vi "Main.vi"() -> ()   [LabVIEW 2020]
uses:
  Userdata.ctl
  <vilib>/drjdpowell/SQLite Library/SQL Connection/Open (string).vi
  <vilib>/drjdpowell/SQLite Library/SQL Connection/Execute SQL (1D String).vi
  <vilib>/drjdpowell/SQLite Library/SQL Connection/Execute SQL (No results).vi
  <vilib>/drjdpowell/SQLite Library/SQL Connection/Connection.lvclass
  <vilib>/drjdpowell/SQLite Library/SQLite.lvlib
panel:
  in  "Tab Control":T1(tab)
  in  "Login":bool
  in  "Password":string
  in  "Username":string
  in  "Exit 2":bool
  out "?":string
  in  "Add User":bool
  in  "Logout":bool
  in  "Exit":bool
  in  "Edit User":bool
  in  "Query User":bool
  in  "Delete User":bool
  in  "Home Add":bool
  in  "Confirm Add":bool
  in  "Userdata_add_page":T2
  out "?":errorcluster
  in  "Home Delete":bool
  in  "Confirm Delete":bool
  in  "Select User to delete":string(combo)
  out "Userdata_delete_page":T2
  in  "Home query":bool
  in  "Select User to more data":string(combo)
  out "Userdata_Query_page":T2
  in  "Home edit":bool
  in  "Confirm Edit":bool
  in  "Select User to Edit":string(combo)
  in  "Userdata_Edit_page":T2
  out "?":errorcluster
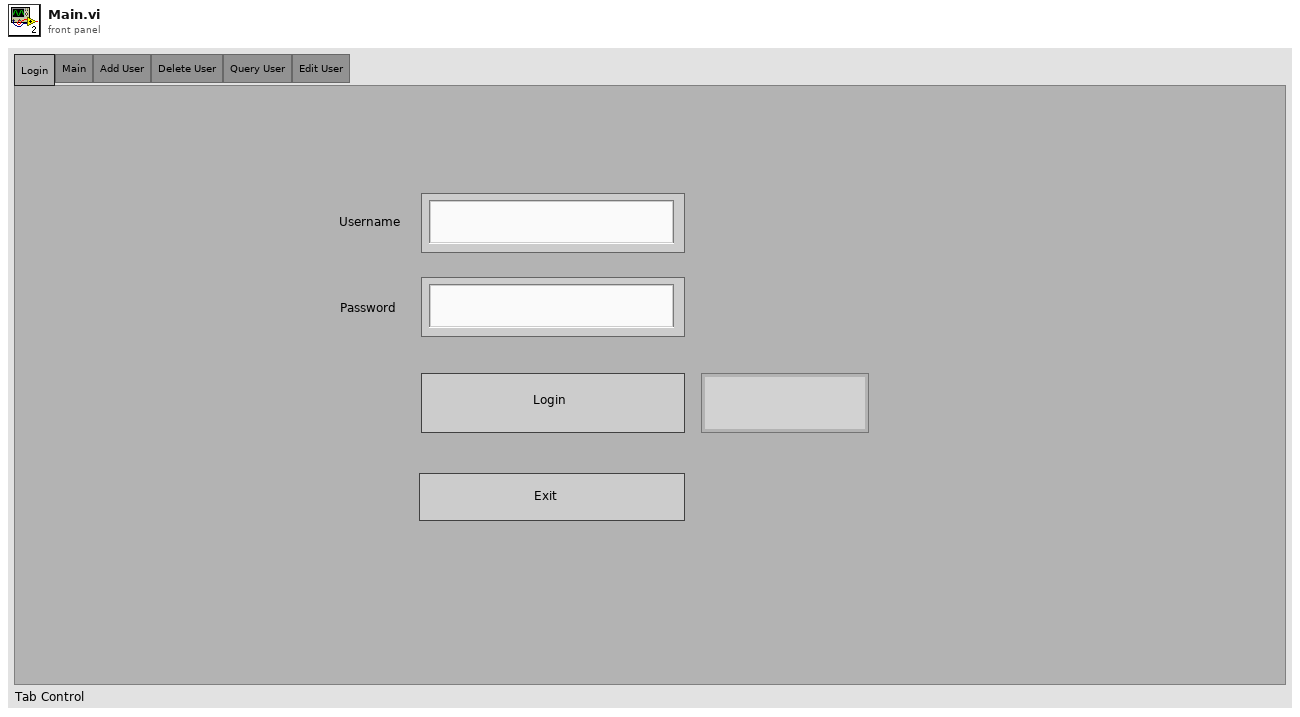
[diagram p1: front panel]
types:
  T1 = enum32{"Login", "Main", "Add User", "Delete User", "Query User", "Edit User"}
  T2 = typedef "Userdata.ctl" = cluster{"Username":string, "Password":string, "Title":string, "Birthdate":timestamp, "Email":string, "User Level":bool}
  T3 = enum32{"Page Enabled", "Page Disabled", "Page Disabled & Grayed"}
  T4 = cluster{"Username":bool, "Password":bool, "Title":bool, "Birthdate":bool, "Email":bool, "User Level":bool}
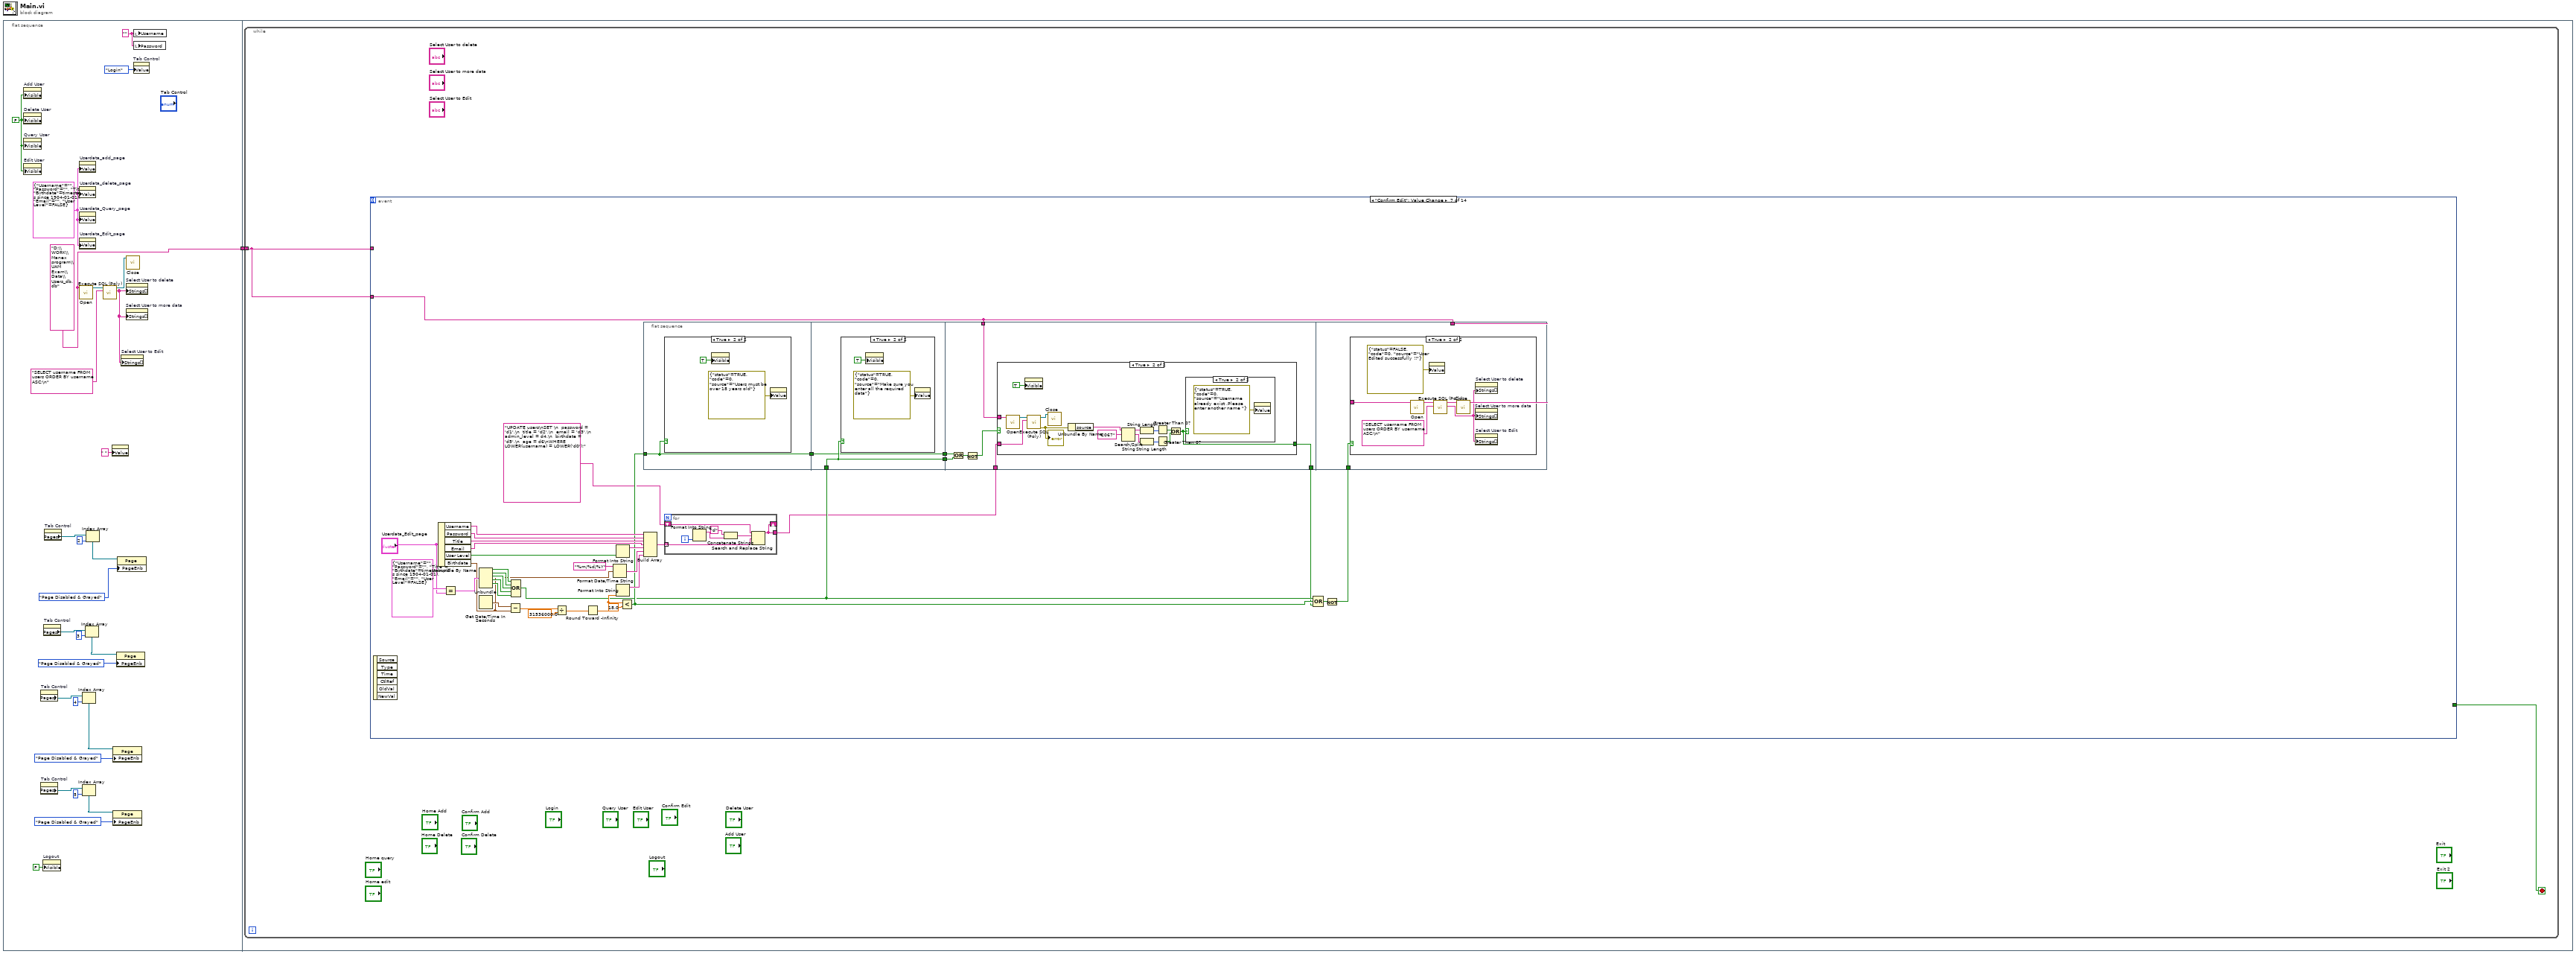
[diagram p0: block diagram]
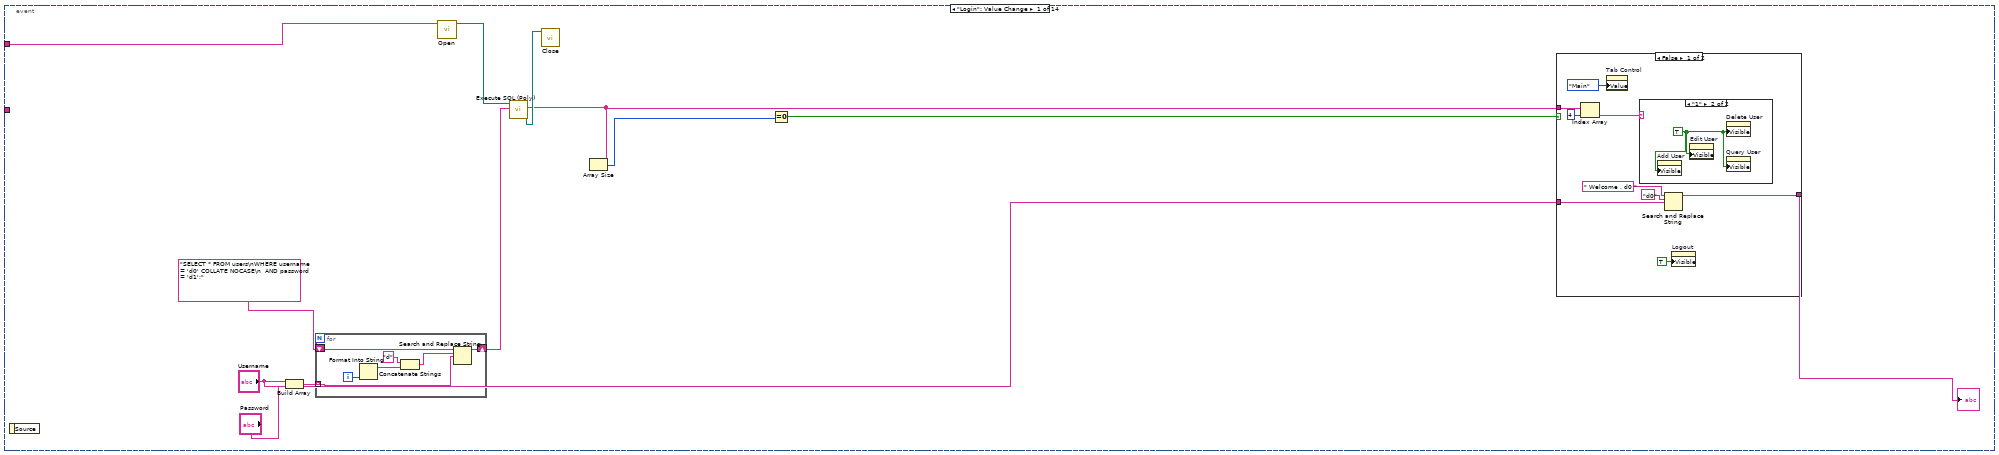
[diagram p2: hidden frame]
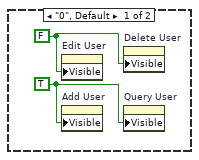
[diagram p3: hidden frame]
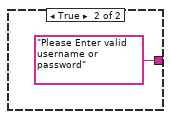
[diagram p4: hidden frame]
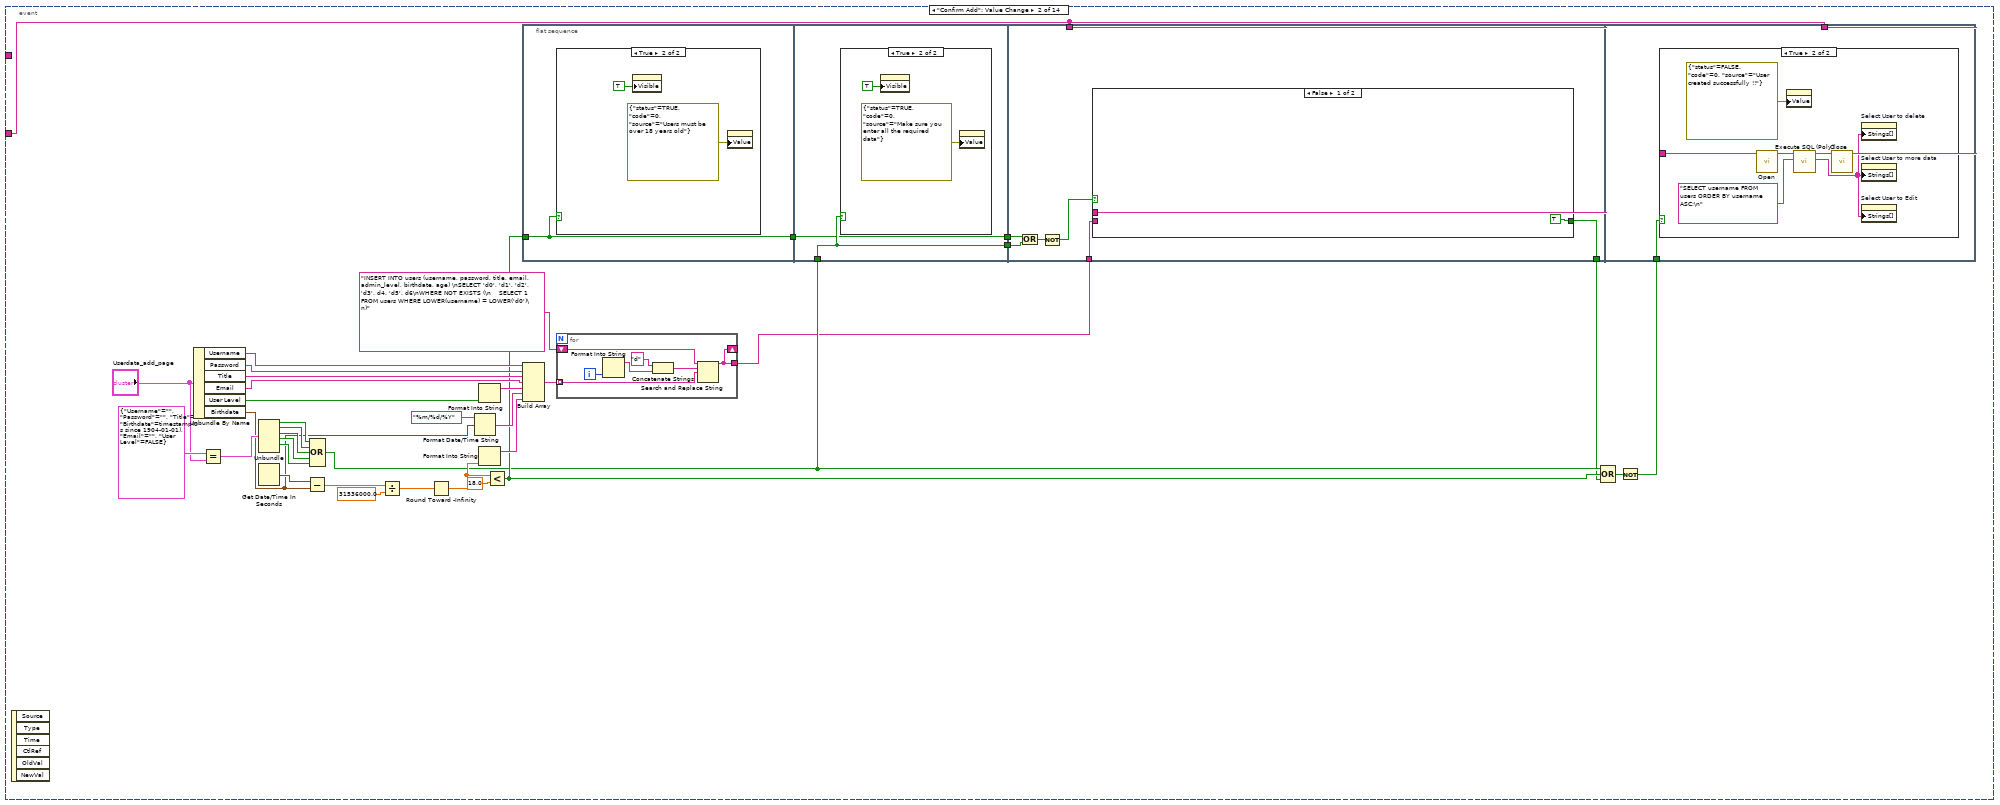
[diagram p5: hidden frame]
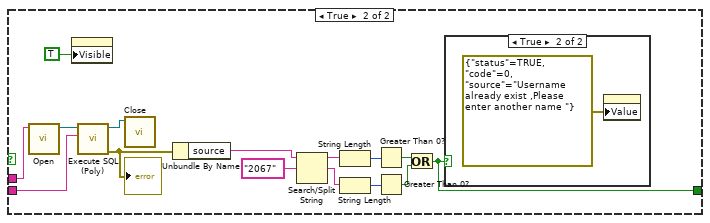
[diagram p8: hidden frame]
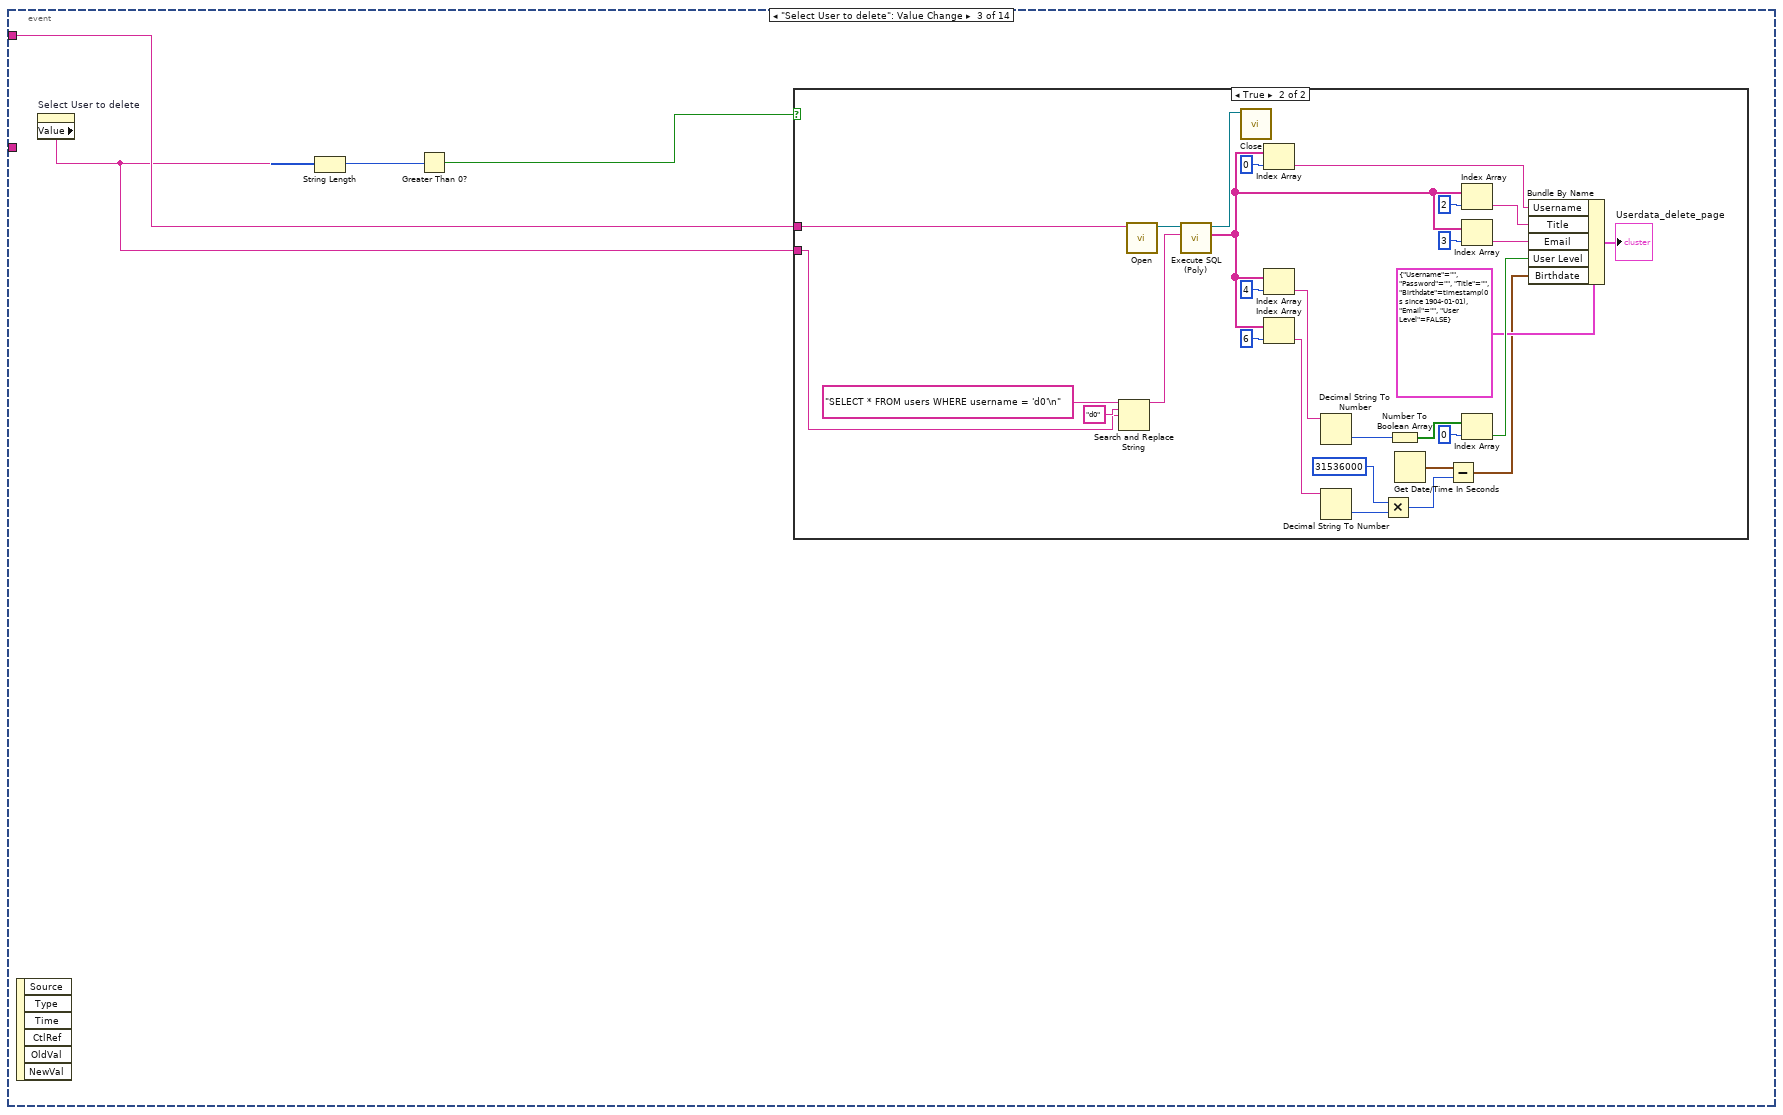
[diagram p11: hidden frame]
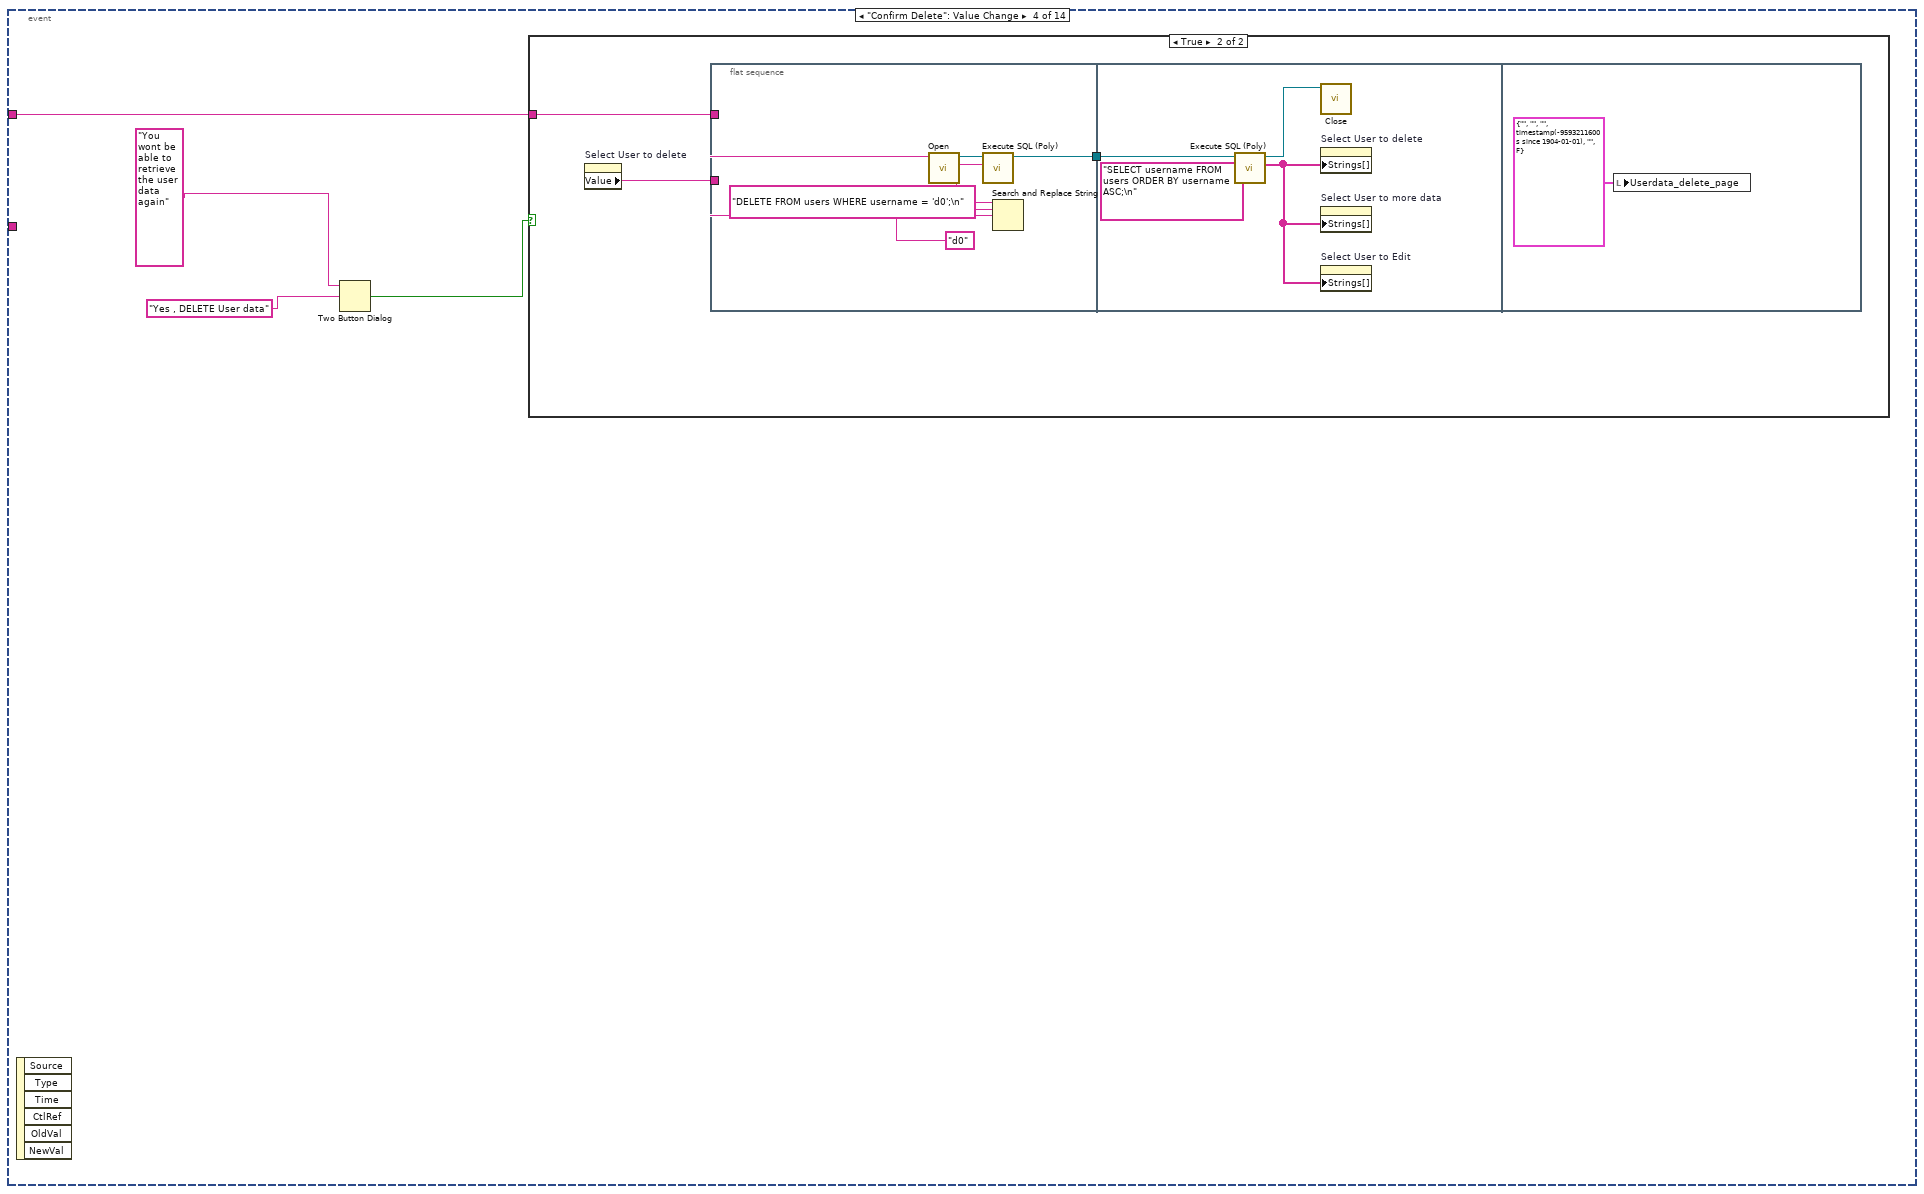
[diagram p13: hidden frame]
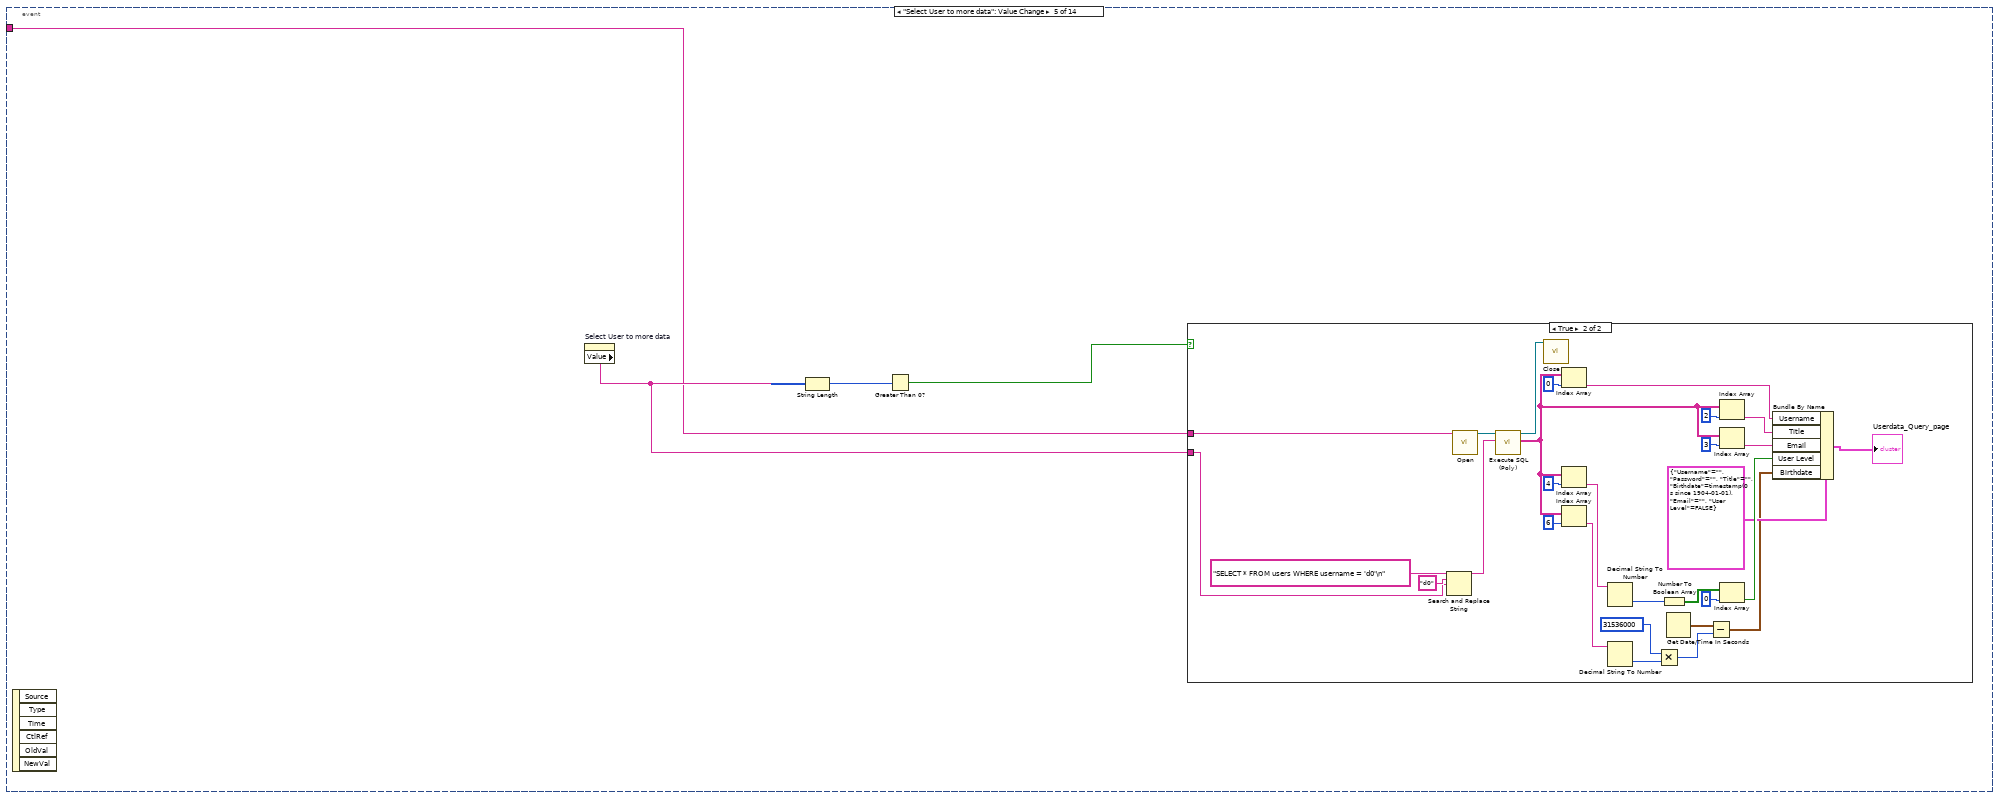
[diagram p15: hidden frame]
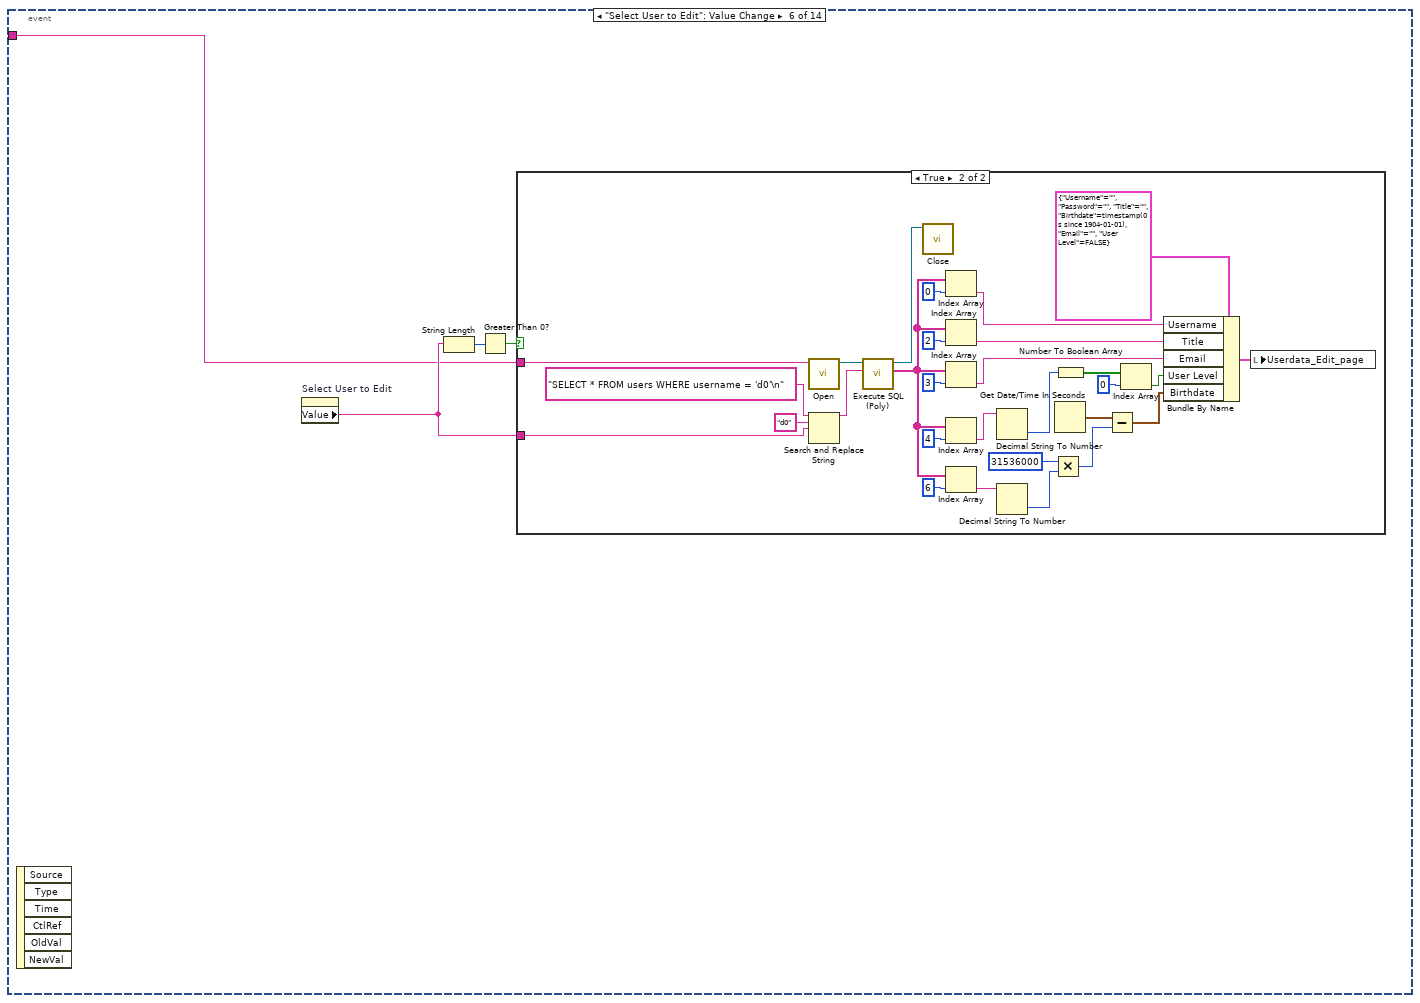
[diagram p17: hidden frame]
diagram:
  n1 = flat-sequence {
    tunnel: [w21] -> w1
    tunnel: w1 -> [w29]
    frame #0 {
      w21 = "D:\\WORK\\Manex program\\UAM Exam\\Data\\Users_db.db" ("db file")
      w25 = T2 {"Username"="", "Password"="", "Title"="", "Birthdate"=timestamp(0 s since 1904-01-01), "Email"="", "User Level"=FALSE} ("Userdata_add_page")
      w26 = FALSE ("Visible")
      w28 = "" ("Username")
      n2 = property on="Add User" class="Bool"("Visible"=w26) -> ()  [unwired: 2 in, 2 out]
      n3 = property on="Delete User" class="Bool"("Visible"=w26) -> ()  [unwired: 2 in, 2 out]
      n4 = property on="Query User" class="Bool"("Visible"=w26) -> ()  [unwired: 2 in, 2 out]
      n5 = property on="Edit User" class="Bool"("Visible"=w26) -> ()  [unwired: 2 in, 2 out]
      n6 = property on="Tab Control" class="TabCtl (strict)"() -> ("Pages"=w11:refnum<vi>[])  [unwired: 2 in, 2 out]
      n7 = property on="Tab Control" class="TabCtl (strict)"() -> ("Pages"=w7:refnum<vi>[])  [unwired: 2 in, 2 out]
      n8 = property on="Logout" class="Bool"("Visible"=FALSE) -> ()  [unwired: 2 in, 2 out]
      n9 = property on="Tab Control" class="TabCtl (strict)"() -> ("Pages"=w15:refnum<vi>[])  [unwired: 2 in, 2 out]
      n10 = property on="Tab Control" class="TabCtl (strict)"() -> ("Pages"=w19:refnum<vi>[])  [unwired: 2 in, 2 out]
      n11 = property on="Userdata_add_page" class="Clust (strict)"("Value"=w25) -> ()  [unwired: 2 in, 2 out]
      n12 = property on="Userdata_delete_page" class="Clust (strict)"("Value"=w25) -> ()  [unwired: 2 in, 2 out]
      n13 = property on="Userdata_Query_page" class="Clust (strict)"("Value"=w25) -> ()  [unwired: 2 in, 2 out]
      n14 = property on="Userdata_Edit_page" class="Clust (strict)"("Value"=w25) -> ()  [unwired: 2 in, 2 out]
      n15 = call-poly <vilib>:"Open.vi"("db file"=w21) -> ("SQLite Connection"=w24:refnum<class "Connection.lvclass">)  [unwired: 9 in, 1 out]
      n16 = Index Array(array=w11, index=4) -> (element=w10:refnum<vi>)
      n17 = Index Array(array=w7, index=5) -> (element=w6:refnum<vi>)
      n18 = Index Array(array=w15, index=3) -> (element=w14:refnum<vi>)
      n19 = Index Array(array=w19, index=2) -> (element=w18:refnum<vi>)
      n20 = call-poly <vilib>:"Execute SQL (Poly).vi"("SQL"="SELECT username FROM users ORDER BY username ASC;\n", "SQLite Connection in"=w24) -> ("Result Set"=w22:string[], "SQLite Connection"=w23:refnum<class "Connection.lvclass">)  [unwired: 6 in, 2 out]
      n21 = property class="Str"("Value"=" ") -> ()  [unwired: 2 in, 2 out]
      n22 = property class="Page"(reference=w10, "PageEnb"=T3."Page Disabled & Grayed" ("Page Enabled State")) -> ()  [unwired: 1 in, 2 out]
      n23 = property class="Page"(reference=w6, "PageEnb"=T3."Page Disabled & Grayed" ("Page Enabled State")) -> ()  [unwired: 1 in, 2 out]
      n24 = property class="Page"(reference=w14, "PageEnb"=T3."Page Disabled & Grayed" ("Page Enabled State")) -> ()  [unwired: 1 in, 2 out]
      n25 = property class="Page"(reference=w18, "PageEnb"=T3."Page Disabled & Grayed" ("Page Enabled State")) -> ()  [unwired: 1 in, 2 out]
      n26 = property on="Select User to Edit" class="CmbBox"("Strings[]"=w22) -> ()  [unwired: 2 in, 2 out]
      n27 = call-dynamic "Close.vi"("SQLite Connection in"=w23) -> ()  [unwired: 10 in, 1 out]
      n28 = property on="Select User to delete" class="CmbBox"("Strings[]"=w22) -> ()  [unwired: 2 in, 2 out]
      n29 = property on="Select User to more data" class="CmbBox"("Strings[]"=w22) -> ()  [unwired: 2 in, 2 out]
      n30 = property on="Tab Control" class="TabCtl (strict)"("Value"=T1."Login" ("Tab Control")) -> ()  [unwired: 2 in, 2 out]
      n31 = local write "Username"(w28) -> ()
      n32 = local write "Password"(w28) -> ()
    }
    frame #1 {
      n33 = while {
        tunnel: w29 -> [w31]
        stop <- w30 stop-if-true
        n34 = event shown="[6] \"Confirm Edit\": Value Change" {
          selector: _ -> [_ _ _ _ _ _ _ _ _ _ _ _ _ _]
          dyn-events: _ -> [_ _ _ _ _ _ _ _ _ _ _ _ _ _]
          timeout: _ -> [_ _ _ _ _ _ _ _ _ _ _ _ _ _]
          tunnel: w31 -> [w36 _ w147 w182 _ _ _ _ _ _ _ _ _ _]
          tunnel: w31 -> [_ w66 _ _ w198 w231 w265 _ _ _ _ _ _ _]
          tunnel: [_ _ _ _ _ _ _ _ _ _ _ _ _ TRUE] -> w30
          event "Login": Value Change {
            n35 = event-data() -> ()  [unwired: 1 in, 1 out]
            n36 = Build Array("Username", "Password") -> (w42:string[])
            n37 = for {
              shift-right: [w62] -> w43
              shift-left: "SELECT * FROM users\nWHERE username = 'd0' COLLATE NOCASE\n  AND password = 'd1';" ("SQL") -> [w63]
              tunnel: w42 -> [w61] mode=indexing
              i -> [w58]
              n38 = Format Into String(w58) -> (resulting string=w60:string)  [unwired: 3 in, 1 out]
              n39 = Concatenate Strings("d" ("string"), w60) -> (w57:string)
              n40 = Search and Replace String(input string=w63, search string=w57, replace string=w61) -> (result string=w62:string)  [unwired: 5 in, 3 out]
            }
            n41 = call-poly <vilib>:"Open.vi"("db file"=w36) -> ("SQLite Connection"=w35:refnum<class "Connection.lvclass">)  [unwired: 9 in, 1 out]
            n42 = call-poly <vilib>:"Execute SQL (Poly).vi"("SQL"=w43, "SQLite Connection in"=w35) -> ("Result Set"=w32:string[], "SQLite Connection"=w37:refnum<class "Connection.lvclass">)  [unwired: 6 in, 2 out]
            n43 = call-dynamic "Close.vi"("SQLite Connection in"=w37) -> ()  [unwired: 10 in, 1 out]
            n44 = Array Size(array=w32) -> (size(s)=w39:i32)
            n45 = Equal To 0?(x=w39) -> (x = 0?=w38:bool)
            n46 = case shown="False" w38 {
              tunnel: "Username" -> [w50 _]
              tunnel: [w49 "Please Enter valid username or password" ("Description")] -> w33
              tunnel: w32 -> [w47 _]
              frame False {
                n47 = Index Array(array=w47, index=4) -> (element=w45:string)
                n48 = property on="Tab Control" class="TabCtl (strict)"("Value"=T1."Main" ("Tab Control")) -> ()  [unwired: 2 in, 2 out]
                n49 = case shown="\"1\"" w45 {
                  frame "0", Default {
                    w54 = FALSE ("Visible")
                    w53 = TRUE ("Visible")
                    n50 = property on="Edit User" class="Bool"("Visible"=w54) -> ()  [unwired: 2 in, 2 out]
                    n51 = property on="Add User" class="Bool"("Visible"=w53) -> ()  [unwired: 2 in, 2 out]
                    n52 = property on="Delete User" class="Bool"("Visible"=w54) -> ()  [unwired: 2 in, 2 out]
                    n53 = property on="Query User" class="Bool"("Visible"=w53) -> ()  [unwired: 2 in, 2 out]
                  }
                  frame "1" {
                    w55 = TRUE ("Visible")
                    n54 = property on="Add User" class="Bool"("Visible"=w55) -> ()  [unwired: 2 in, 2 out]
                    n55 = property on="Edit User" class="Bool"("Visible"=w55) -> ()  [unwired: 2 in, 2 out]
                    n56 = property on="Delete User" class="Bool"("Visible"=w55) -> ()  [unwired: 2 in, 2 out]
                    n57 = property on="Query User" class="Bool"("Visible"=w55) -> ()  [unwired: 2 in, 2 out]
                  }
                }
                n58 = Search and Replace String(input string=" Welcome , d0 " ("Description"), search string="d0", replace string=w50) -> (result string=w49:string)  [unwired: 5 in, 3 out]
                n59 = property on="Logout" class="Bool"("Visible"=TRUE) -> ()  [unwired: 2 in, 2 out]
              }
              frame True {
              }
            }
            "?" <- w33
          }
          event "Confirm Add": Value Change {
            n60 = event-data() -> ()  [unwired: 1 in, 6 out]
            n61 = Unbundle By Name("Userdata_add_page") -> ("Username"=w81:string, "Password"=w80:string, "Title"=w79:string, "Email"=w78:string, "User Level"=w77:bool, "Birthdate"=w76:timestamp)
            n62 = Equal?(x=T2 {"Username"="", "Password"="", "Title"="", "Birthdate"=timestamp(0 s since 1904-01-01), "Email"="", "User Level"=FALSE} ("Userdata_add_page"), y="Userdata_add_page") -> (x = y?=w82:T4)
            n63 = Unbundle(w82) -> ("Username"=w84:bool, "Password"=w85:bool, "Title"=w86:bool, "Birthdate"=w87:bool, "Email"=w88:bool)  [unwired: 1 out]
            n64 = Get Date/Time In Seconds() -> (seconds since 1Jan1904=w95:timestamp)
            n65 = Subtract(x=w95, y=w76) -> (x-y=w72:dbl)
            n66 = Compound Arithmetic op=OR(w84, w85, w86, w87, w88) -> (w70:bool)
            n67 = Divide(x=w72, y=31536000.0) -> (x/y=w99:dbl)
            n68 = Round Toward -Infinity(1:w99) -> (0:w90:dbl)
            n69 = Format Date/Time String(time format string (%c)="%m/%d/%Y", seconds (now)=w76) -> (date/time string=w94:string)  [unwired: 1 in]
            n70 = Format Into String(w77) -> (resulting string=w98:string)  [unwired: 3 in, 1 out]
            n71 = Format Into String(w90) -> (resulting string=w96:string)  [unwired: 3 in, 1 out]
            n72 = Less?(x=w90, y=18.0) -> (x < y?=w71:bool)
            n73 = flat-sequence {
              tunnel: w71 -> [w100]
              tunnel: [w100] -> w68
              tunnel: w70 -> [w104]
              tunnel: [w104] -> w69
              tunnel: w68 -> [w103]
              tunnel: [w103] -> w67
              tunnel: w66 -> [w113]
              tunnel: w69 -> [w110]
              tunnel: w67 -> [w109]
              tunnel: [w108] -> w65
              tunnel: w64 -> [w107]
              tunnel: w73 -> [w132]
              tunnel: w66 -> [w131]
              frame #0 {
                n74 = case shown="True" w100 {
                  frame False {
                  }
                  frame True {
                    n75 = property class="Clust (strict)"("Visible"=TRUE) -> ()  [unwired: 2 in, 2 out]
                    n76 = property class="Clust (strict)"("Value"=errorcluster {"status"=TRUE, "code"=0, "source"="Users must be over 18 years old"} ("error out")) -> ()  [unwired: 2 in, 2 out]
                  }
                }
              }
              frame #1 {
                n77 = case shown="True" w104 {
                  frame False {
                  }
                  frame True {
                    n78 = property class="Clust (strict)"("Visible"=TRUE) -> ()  [unwired: 2 in, 2 out]
                    n79 = property class="Clust (strict)"("Value"=errorcluster {"status"=TRUE, "code"=0, "source"="Make sure you enter all the required data"} ("error out")) -> ()  [unwired: 2 in, 2 out]
                  }
                }
              }
              frame #2 {
                n80 = Or(x=w109, y=w110) -> (x .or. y?=w112:bool)
                n81 = Not(x=w112) -> (.not. x?=w111:bool)
                n82 = case shown="False" w111 {
                  tunnel: w113 -> [_ w118]
                  tunnel: [TRUE w116] -> w108
                  tunnel: w107 -> [_ w115]
                  frame False {
                  }
                  frame True {
                    n83 = call-poly <vilib>:"Open.vi"("db file"=w118) -> ("SQLite Connection"=w127:refnum<class "Connection.lvclass">)  [unwired: 9 in, 1 out]
                    n84 = property class="Clust (strict)"("Visible"=TRUE) -> ()  [unwired: 2 in, 2 out]
                    n85 = call-poly <vilib>:"Execute SQL (Poly).vi"("SQL"=w115, "SQLite Connection in"=w127) -> ("error out"=w120:errorcluster, "SQLite Connection"=w117:refnum<class "Connection.lvclass">)  [unwired: 8 in]
                    "?" <- w120
                    n86 = call-dynamic "Close.vi"("SQLite Connection in"=w117) -> ()  [unwired: 10 in, 1 out]
                    n87 = Unbundle By Name(w120) -> ("source"=w121:string)
                    n88 = Search/Split String(string=w121, search string/char (-)="2067") -> (substring before match=w128:string, match + rest of string=w122:string)  [unwired: 1 in, 1 out]
                    n89 = String Length(string=w128) -> (length=w123:i32)
                    n90 = String Length(string=w122) -> (length=w125:i32)
                    n91 = Greater Than 0?(x=w123) -> (x > 0?=w124:bool)
                    n92 = Greater Than 0?(x=w125) -> (x > 0?=w126:bool)
                    n93 = Or(x=w124, y=w126) -> (x .or. y?=w116:bool)
                    n94 = case shown="True" w116 {
                      frame False {
                      }
                      frame True {
                        n95 = property class="Clust (strict)"("Value"=errorcluster {"status"=TRUE, "code"=0, "source"="Username already exist ,Please enter another name "} ("error out")) -> ()  [unwired: 2 in, 2 out]
                      }
                    }
                  }
                }
              }
              frame #3 {
                n96 = case shown="True" w132 {
                  tunnel: w131 -> [_ w133]
                  frame False {
                  }
                  frame True {
                    n97 = call-poly <vilib>:"Open.vi"("db file"=w133) -> ("SQLite Connection"=w134:refnum<class "Connection.lvclass">)  [unwired: 9 in, 1 out]
                    n98 = property class="Clust (strict)"("Value"=errorcluster {"status"=FALSE, "code"=0, "source"="User created successfully !!"} ("error out")) -> ()  [unwired: 2 in, 2 out]
                    n99 = call-poly <vilib>:"Execute SQL (Poly).vi"("SQL"="SELECT username FROM users ORDER BY username ASC;\n", "SQLite Connection in"=w134) -> ("Result Set"=w137:string[], "SQLite Connection"=w136:refnum<class "Connection.lvclass">)  [unwired: 6 in, 2 out]
                    n100 = call-dynamic "Close.vi"("SQLite Connection in"=w136) -> ()  [unwired: 10 in, 1 out]
                    n101 = property on="Select User to delete" class="CmbBox"("Strings[]"=w137) -> ()  [unwired: 2 in, 2 out]
                    n102 = property on="Select User to more data" class="CmbBox"("Strings[]"=w137) -> ()  [unwired: 2 in, 2 out]
                    n103 = property on="Select User to Edit" class="CmbBox"("Strings[]"=w137) -> ()  [unwired: 2 in, 2 out]
                  }
                }
              }
            }
            n104 = Build Array(w81, w80, w79, w78, w98, w94, w96) -> (w97:string[])
            n105 = for {
              tunnel: w97 -> [w140] mode=indexing
              tunnel: [w139] -> w64
              shift-right: [w139] -> _
              shift-left: "INSERT INTO users (username, password, title, email, admin_level, birthdate, age) \nSELECT 'd0', 'd1', 'd2', 'd3', d4, 'd5', d6\nWHERE NOT EXISTS (\n    SELECT 1 FROM users WHERE LOWER(username) = LOWER('d0')\n)" ("string") -> [w142]
              i -> [w145]
              n106 = Format Into String(w145) -> (resulting string=w144:string)  [unwired: 3 in, 1 out]
              n107 = Concatenate Strings("d" ("string"), w144) -> (w141:string)
              n108 = Search and Replace String(input string=w142, search string=w141, replace string=w140) -> (result string=w139:string)  [unwired: 5 in, 3 out]
            }
            n109 = Compound Arithmetic op=OR(w70, w71, w65) -> (w74:bool)
            n110 = Not(x=w74) -> (.not. x?=w73:bool)
          }
          event "Select User to delete": Value Change {
            n111 = event-data() -> ()  [unwired: 1 in, 6 out]
            n112 = property on="Select User to delete" class="CmbBox"() -> ("Value"=w146:string)  [unwired: 2 in, 2 out]
            n113 = String Length(string=w146) -> (length=w149:i32)
            n114 = Greater Than 0?(x=w149) -> (x > 0?=w148:bool)
            n115 = case shown="True" w148 {
              tunnel: w147 -> [_ w174]
              tunnel: w146 -> [_ w173]
              frame False {
              }
              frame True {
                n116 = Search and Replace String(input string="SELECT * FROM users WHERE username = 'd0'\n" ("SQL"), search string="d0", replace string=w173) -> (result string=w171:string)  [unwired: 5 in, 3 out]
                n117 = call-poly <vilib>:"Open.vi"("db file"=w174) -> ("SQLite Connection"=w177:refnum<class "Connection.lvclass">)  [unwired: 9 in, 1 out]
                n118 = call-poly <vilib>:"Execute SQL (Poly).vi"("SQL"=w171, "SQLite Connection in"=w177) -> ("Result Set"=w172:string[], "SQLite Connection"=w178:refnum<class "Connection.lvclass">)  [unwired: 6 in, 2 out]
                n119 = call-dynamic "Close.vi"("SQLite Connection in"=w178) -> ()  [unwired: 10 in, 1 out]
                n120 = Index Array(array=w172, index=0) -> (element=w162:string)
                n121 = Index Array(array=w172, index=4) -> (element=w170:string)
                n122 = Index Array(array=w172, index=6) -> (element=w166:string)
                n123 = Decimal String To Number(string=w170) -> (number=w167:i32)  [unwired: 2 in, 1 out]
                n124 = Decimal String To Number(string=w166) -> (number=w161:i32)  [unwired: 2 in, 1 out]
                n125 = Multiply(x=31536000, y=w161) -> (x*y=w151:i32)
                n126 = Number To Boolean Array(number=w167) -> (Boolean array=w168:bool[])
                n127 = Get Date/Time In Seconds() -> (seconds since 1Jan1904=w152:timestamp)
                n128 = Subtract(x=w152, y=w151) -> (x-y=w150:timestamp)
                n129 = Index Array(array=w172, index=2) -> (element=w164:string)
                n130 = Index Array(array=w172, index=3) -> (element=w165:string)
                n131 = Index Array(array=w168, index=0) -> (element=w169:bool)
                n132 = Bundle By Name(cluster=T2 {"Username"="", "Password"="", "Title"="", "Birthdate"=timestamp(0 s since 1904-01-01), "Email"="", "User Level"=FALSE} ("Userdata_delete_page"), "Username"=w162, "Title"=w164, "Email"=w165, "User Level"=w169, "Birthdate"=w150) -> (→"Userdata_delete_page":T2)
              }
            }
          }
          event "Confirm Delete": Value Change {
            n133 = event-data() -> ()  [unwired: 1 in, 6 out]
            n134 = Two Button Dialog(message="You wont be able to retrieve the user data again", 2:"Yes , DELETE User data" ("T button name (\"OK\")")) -> (T button?=w180:bool)  [unwired: 1 in]
            n135 = case shown="True" w180 {
              tunnel: w182 -> [_ w184]
              frame False {
              }
              frame True {
                n136 = property on="Select User to delete" class="CmbBox"() -> ("Value"=w183:string)  [unwired: 2 in, 2 out]
                n137 = flat-sequence {
                  tunnel: w183 -> [w191]
                  tunnel: w184 -> [w188]
                  tunnel: [w186] -> w185
                  tunnel: w185 -> [w193]
                  frame #0 {
                    n138 = call-poly <vilib>:"Open.vi"("db file"=w188) -> ("SQLite Connection"=w189:refnum<class "Connection.lvclass">)  [unwired: 9 in, 1 out]
                    n139 = Search and Replace String(input string="DELETE FROM users WHERE username = 'd0';\n", search string="d0", replace string=w191) -> (result string=w187:string)  [unwired: 5 in, 3 out]
                    n140 = call-poly <vilib>:"Execute SQL (Poly).vi"("SQL"=w187, "SQLite Connection in"=w189) -> ("SQLite Connection"=w186:refnum<class "Connection.lvclass">)  [unwired: 6 in, 3 out]
                  }
                  frame #1 {
                    n141 = call-poly <vilib>:"Execute SQL (Poly).vi"("SQL"="SELECT username FROM users ORDER BY username ASC;\n", "SQLite Connection in"=w193) -> ("Result Set"=w195:string[], "SQLite Connection"=w196:refnum<class "Connection.lvclass">)  [unwired: 6 in, 2 out]
                    n142 = call-dynamic "Close.vi"("SQLite Connection in"=w196) -> ()  [unwired: 10 in, 1 out]
                    n143 = property on="Select User to delete" class="CmbBox"("Strings[]"=w195) -> ()  [unwired: 2 in, 2 out]
                    n144 = property on="Select User to more data" class="CmbBox"("Strings[]"=w195) -> ()  [unwired: 2 in, 2 out]
                    n145 = property on="Select User to Edit" class="CmbBox"("Strings[]"=w195) -> ()  [unwired: 2 in, 2 out]
                  }
                  frame #2 {
                    n146 = local write "Userdata_delete_page"(T2 {"Username"="", "Password"="", "Title"="", "Birthdate"=timestamp(-9593211600 s since 1904-01-01), "Email"="", "User Level"=FALSE} ("Userdata_delete_page")) -> ()
                  }
                }
              }
            }
          }
          event "Select User to more data": Value Change {
            n147 = event-data() -> ()  [unwired: 1 in, 6 out]
            n148 = property on="Select User to more data" class="CmbBox"() -> ("Value"=w199:string)  [unwired: 2 in, 2 out]
            n149 = String Length(string=w199) -> (length=w201:i32)
            n150 = Greater Than 0?(x=w201) -> (x > 0?=w200:bool)
            n151 = case shown="True" w200 {
              tunnel: w198 -> [_ w226]
              tunnel: w199 -> [_ w225]
              frame False {
              }
              frame True {
                n152 = Search and Replace String(input string="SELECT * FROM users WHERE username = 'd0'\n" ("SQL"), search string="d0", replace string=w225) -> (result string=w223:string)  [unwired: 5 in, 3 out]
                n153 = call-poly <vilib>:"Open.vi"("db file"=w226) -> ("SQLite Connection"=w229:refnum<class "Connection.lvclass">)  [unwired: 9 in, 1 out]
                n154 = call-poly <vilib>:"Execute SQL (Poly).vi"("SQL"=w223, "SQLite Connection in"=w229) -> ("Result Set"=w224:string[], "SQLite Connection"=w230:refnum<class "Connection.lvclass">)  [unwired: 6 in, 2 out]
                n155 = call-dynamic "Close.vi"("SQLite Connection in"=w230) -> ()  [unwired: 10 in, 1 out]
                n156 = Index Array(array=w224, index=0) -> (element=w215:string)
                n157 = Index Array(array=w224, index=4) -> (element=w222:string)
                n158 = Index Array(array=w224, index=6) -> (element=w218:string)
                n159 = Decimal String To Number(string=w222) -> (number=w219:i32)  [unwired: 2 in, 1 out]
                n160 = Decimal String To Number(string=w218) -> (number=w214:i32)  [unwired: 2 in, 1 out]
                n161 = Multiply(x=31536000, y=w214) -> (x*y=w204:i32)
                n162 = Number To Boolean Array(number=w219) -> (Boolean array=w220:bool[])
                n163 = Get Date/Time In Seconds() -> (seconds since 1Jan1904=w205:timestamp)
                n164 = Subtract(x=w205, y=w204) -> (x-y=w203:timestamp)
                n165 = Index Array(array=w224, index=2) -> (element=w216:string)
                n166 = Index Array(array=w224, index=3) -> (element=w217:string)
                n167 = Index Array(array=w220, index=0) -> (element=w221:bool)
                n168 = Bundle By Name(cluster=T2 {"Username"="", "Password"="", "Title"="", "Birthdate"=timestamp(0 s since 1904-01-01), "Email"="", "User Level"=FALSE} ("Userdata_delete_page"), "Username"=w215, "Title"=w216, "Email"=w217, "User Level"=w221, "Birthdate"=w203) -> (→"Userdata_Query_page":T2)
              }
            }
          }
          event "Select User to Edit": Value Change {
            n169 = event-data() -> ()  [unwired: 1 in, 6 out]
            n170 = property on="Select User to Edit" class="CmbBox"() -> ("Value"=w232:string)  [unwired: 2 in, 2 out]
            n171 = String Length(string=w232) -> (length=w234:i32)
            n172 = Greater Than 0?(x=w234) -> (x > 0?=w233:bool)
            n173 = case shown="True" w233 {
              tunnel: w231 -> [_ w259]
              tunnel: w232 -> [_ w258]
              frame False {
              }
              frame True {
                n174 = call-poly <vilib>:"Open.vi"("db file"=w259) -> ("SQLite Connection"=w262:refnum<class "Connection.lvclass">)  [unwired: 9 in, 1 out]
                n175 = Search and Replace String(input string="SELECT * FROM users WHERE username = 'd0'\n" ("SQL"), search string="d0", replace string=w258) -> (result string=w256:string)  [unwired: 5 in, 3 out]
                n176 = call-poly <vilib>:"Execute SQL (Poly).vi"("SQL"=w256, "SQLite Connection in"=w262) -> ("Result Set"=w257:string[], "SQLite Connection"=w263:refnum<class "Connection.lvclass">)  [unwired: 6 in, 2 out]
                n177 = call-dynamic "Close.vi"("SQLite Connection in"=w263) -> ()  [unwired: 10 in, 1 out]
                n178 = Index Array(array=w257, index=0) -> (element=w248:string)
                n179 = Index Array(array=w257, index=2) -> (element=w249:string)
                n180 = Index Array(array=w257, index=3) -> (element=w250:string)
                n181 = Index Array(array=w257, index=4) -> (element=w255:string)
                n182 = Index Array(array=w257, index=6) -> (element=w251:string)
                n183 = Decimal String To Number(string=w255) -> (number=w252:i32)  [unwired: 2 in, 1 out]
                n184 = Decimal String To Number(string=w251) -> (number=w247:i32)  [unwired: 2 in, 1 out]
                n185 = Multiply(x=31536000, y=w247) -> (x*y=w237:i32)
                n186 = Get Date/Time In Seconds() -> (seconds since 1Jan1904=w238:timestamp)
                n187 = Number To Boolean Array(number=w252) -> (Boolean array=w253:bool[])
                n188 = Subtract(x=w238, y=w237) -> (x-y=w236:timestamp)
                n189 = Index Array(array=w253, index=0) -> (element=w254:bool)
                n190 = Bundle By Name(cluster=T2 {"Username"="", "Password"="", "Title"="", "Birthdate"=timestamp(0 s since 1904-01-01), "Email"="", "User Level"=FALSE} ("Userdata_delete_page"), "Username"=w248, "Title"=w249, "Email"=w250, "User Level"=w254, "Birthdate"=w236) -> (w235:T2)
                n191 = local write "Userdata_Edit_page"(w235) -> ()
              }
            }
          }
          event "Confirm Edit": Value Change {
            n192 = event-data() -> ()  [unwired: 1 in, 6 out]
            n193 = Unbundle By Name("Userdata_Edit_page") -> ("Username"=w279:string, "Password"=w278:string, "Title"=w277:string, "Email"=w276:string, "User Level"=w275:bool, "Birthdate"=w274:timestamp)
            n194 = Equal?(x=T2 {"Username"="", "Password"="", "Title"="", "Birthdate"=timestamp(0 s since 1904-01-01), "Email"="", "User Level"=FALSE} ("Userdata_add_page"), y="Userdata_Edit_page") -> (x = y?=w280:T4)
            n195 = Unbundle(w280) -> ("Username"=w282:bool, "Password"=w283:bool, "Title"=w284:bool, "Birthdate"=w285:bool, "Email"=w286:bool)  [unwired: 1 out]
            n196 = Get Date/Time In Seconds() -> (seconds since 1Jan1904=w292:timestamp)
            n197 = Subtract(x=w292, y=w274) -> (x-y=w271:dbl)
            n198 = Compound Arithmetic op=OR(w282, w283, w284, w285, w286) -> (w269:bool)
            n199 = Divide(x=w271, y=31536000.0) -> (x/y=w296:dbl)
            n200 = Round Toward -Infinity(1:w296) -> (0:w288:dbl)
            n201 = Format Date/Time String(time format string (%c)="%m/%d/%Y", seconds (now)=w274) -> (date/time string=w291:string)  [unwired: 1 in]
            n202 = Format Into String(w275) -> (resulting string=w295:string)  [unwired: 3 in, 1 out]
            n203 = Format Into String(w288) -> (resulting string=w293:string)  [unwired: 3 in, 1 out]
            n204 = Less?(x=w288, y=18.0) -> (x < y?=w270:bool)
            n205 = flat-sequence {
              tunnel: w270 -> [w300]
              tunnel: [w300] -> w299
              tunnel: w269 -> [w304]
              tunnel: [w304] -> w298
              tunnel: w299 -> [w303]
              tunnel: [w303] -> w297
              tunnel: w265 -> [w307]
              tunnel: w298 -> [w311]
              tunnel: w297 -> [w310]
              tunnel: [w309] -> w268
              tunnel: w267 -> [w308]
              tunnel: w272 -> [w332]
              tunnel: w265 -> [w331]
              frame #0 {
                n206 = case shown="True" w300 {
                  frame False {
                  }
                  frame True {
                    n207 = property class="Clust (strict)"("Visible"=TRUE) -> ()  [unwired: 2 in, 2 out]
                    n208 = property class="Clust (strict)"("Value"=errorcluster {"status"=TRUE, "code"=0, "source"="Users must be over 18 years old"} ("error out")) -> ()  [unwired: 2 in, 2 out]
                  }
                }
              }
              frame #1 {
                n209 = case shown="True" w304 {
                  frame False {
                  }
                  frame True {
                    n210 = property class="Clust (strict)"("Visible"=TRUE) -> ()  [unwired: 2 in, 2 out]
                    n211 = property class="Clust (strict)"("Value"=errorcluster {"status"=TRUE, "code"=0, "source"="Make sure you enter all the required data"} ("error out")) -> ()  [unwired: 2 in, 2 out]
                  }
                }
              }
              frame #2 {
                n212 = Or(x=w310, y=w311) -> (x .or. y?=w313:bool)
                n213 = Not(x=w313) -> (.not. x?=w312:bool)
                n214 = case shown="True" w312 {
                  tunnel: [TRUE w317] -> w309
                  tunnel: w308 -> [_ w316]
                  tunnel: w307 -> [_ w315]
                  frame False {
                  }
                  frame True {
                    n215 = call-poly <vilib>:"Open.vi"("db file"=w315) -> ("SQLite Connection"=w327:refnum<class "Connection.lvclass">)  [unwired: 9 in, 1 out]
                    n216 = property class="Clust (strict)"("Visible"=TRUE) -> ()  [unwired: 2 in, 2 out]
                    n217 = call-poly <vilib>:"Execute SQL (Poly).vi"("SQL"=w316, "SQLite Connection in"=w327) -> ("error out"=w320:errorcluster, "SQLite Connection"=w318:refnum<class "Connection.lvclass">)  [unwired: 8 in]
                    "?" <- w320
                    n218 = call-dynamic "Close.vi"("SQLite Connection in"=w318) -> ()  [unwired: 10 in, 1 out]
                    n219 = Unbundle By Name(w320) -> ("source"=w321:string)
                    n220 = Search/Split String(string=w321, search string/char (-)="2067") -> (substring before match=w328:string, match + rest of string=w322:string)  [unwired: 1 in, 1 out]
                    n221 = String Length(string=w328) -> (length=w323:i32)
                    n222 = String Length(string=w322) -> (length=w325:i32)
                    n223 = Greater Than 0?(x=w323) -> (x > 0?=w324:bool)
                    n224 = Greater Than 0?(x=w325) -> (x > 0?=w326:bool)
                    n225 = Or(x=w324, y=w326) -> (x .or. y?=w317:bool)
                    n226 = case shown="True" w317 {
                      frame False {
                      }
                      frame True {
                        n227 = property class="Clust (strict)"("Value"=errorcluster {"status"=TRUE, "code"=0, "source"="Username already exist ,Please enter another name "} ("error out")) -> ()  [unwired: 2 in, 2 out]
                      }
                    }
                  }
                }
              }
              frame #3 {
                n228 = case shown="True" w332 {
                  tunnel: w331 -> [_ w333]
                  frame False {
                  }
                  frame True {
                    n229 = call-poly <vilib>:"Open.vi"("db file"=w333) -> ("SQLite Connection"=w334:refnum<class "Connection.lvclass">)  [unwired: 9 in, 1 out]
                    n230 = property class="Clust (strict)"("Value"=errorcluster {"status"=FALSE, "code"=0, "source"="User Edited successfully !!"} ("error out")) -> ()  [unwired: 2 in, 2 out]
                    n231 = call-poly <vilib>:"Execute SQL (Poly).vi"("SQL"="SELECT username FROM users ORDER BY username ASC;\n", "SQLite Connection in"=w334) -> ("Result Set"=w337:string[], "SQLite Connection"=w336:refnum<class "Connection.lvclass">)  [unwired: 6 in, 2 out]
                    n232 = call-dynamic "Close.vi"("SQLite Connection in"=w336) -> ()  [unwired: 10 in, 1 out]
                    n233 = property on="Select User to delete" class="CmbBox"("Strings[]"=w337) -> ()  [unwired: 2 in, 2 out]
                    n234 = property on="Select User to more data" class="CmbBox"("Strings[]"=w337) -> ()  [unwired: 2 in, 2 out]
                    n235 = property on="Select User to Edit" class="CmbBox"("Strings[]"=w337) -> ()  [unwired: 2 in, 2 out]
                  }
                }
              }
            }
            n236 = Build Array(w279, w278, w277, w276, w295, w291, w293) -> (w294:string[])
            n237 = for {
              tunnel: w294 -> [w340] mode=indexing
              tunnel: [w339] -> w267
              shift-right: [w339] -> _
              shift-left: "UPDATE users\nSET \n  password = 'd1',\n  title = 'd2',\n  email = 'd3',\n  admin_level = d4,\n  birthdate = 'd5',\n  age = d6\nWHERE LOWER(username) = LOWER('d0');" ("string") -> [w342]
              i -> [w345]
              n238 = Format Into String(w345) -> (resulting string=w344:string)  [unwired: 3 in, 1 out]
              n239 = Concatenate Strings("d" ("string"), w344) -> (w341:string)
              n240 = Search and Replace String(input string=w342, search string=w341, replace string=w340) -> (result string=w339:string)  [unwired: 5 in, 3 out]
            }
            n241 = Compound Arithmetic op=OR(w269, w270, w268) -> (w273:bool)
            n242 = Not(x=w273) -> (.not. x?=w272:bool)
          }
          event "Home Add", "Home Delete", "Home query", "Home edit": Value Change {
            n243 = event-data() -> ()  [unwired: 1 in, 6 out]
            n244 = property on="Tab Control" class="TabCtl (strict)"("Value"=T1."Main" ("Tab Control")) -> ()  [unwired: 2 in, 2 out]
          }
          event "Logout": Value Change {
            w365 = FALSE ("Visible")
            w366 = "" ("Username")
            n245 = event-data() -> ()  [unwired: 1 in, 6 out]
            n246 = local write "Password"(w366) -> ()
            n247 = local write "Username"(w366) -> ()
            n248 = property on="Tab Control" class="TabCtl (strict)"("Value"=T1."Login" ("Tab Control")) -> ()  [unwired: 2 in, 2 out]
            n249 = property on="Query User" class="Bool"("Visible"=w365) -> ()  [unwired: 2 in, 2 out]
            n250 = property on="Delete User" class="Bool"("Visible"=w365) -> ()  [unwired: 2 in, 2 out]
            n251 = property on="Edit User" class="Bool"("Visible"=w365) -> ()  [unwired: 2 in, 2 out]
            n252 = property on="Logout" class="Bool"("Visible"=FALSE) -> ()  [unwired: 2 in, 2 out]
            n253 = property on="Add User" class="Bool"("Visible"=w365) -> ()  [unwired: 2 in, 2 out]
            n254 = property on="Tab Control" class="TabCtl (strict)"() -> ("Pages"=w356:refnum<vi>[])  [unwired: 2 in, 2 out]
            n255 = property on="Tab Control" class="TabCtl (strict)"() -> ("Pages"=w352:refnum<vi>[])  [unwired: 2 in, 2 out]
            n256 = property on="Tab Control" class="TabCtl (strict)"() -> ("Pages"=w360:refnum<vi>[])  [unwired: 2 in, 2 out]
            n257 = property on="Tab Control" class="TabCtl (strict)"() -> ("Pages"=w364:refnum<vi>[])  [unwired: 2 in, 2 out]
            n258 = Index Array(array=w356, index=4) -> (element=w355:refnum<vi>)
            n259 = Index Array(array=w352, index=5) -> (element=w351:refnum<vi>)
            n260 = Index Array(array=w360, index=3) -> (element=w359:refnum<vi>)
            n261 = Index Array(array=w364, index=2) -> (element=w363:refnum<vi>)
            n262 = property class="Page"(reference=w355, "PageEnb"=T3."Page Disabled & Grayed" ("Page Enabled State")) -> ()  [unwired: 1 in, 2 out]
            n263 = property class="Page"(reference=w351, "PageEnb"=T3."Page Disabled & Grayed" ("Page Enabled State")) -> ()  [unwired: 1 in, 2 out]
            n264 = property class="Page"(reference=w359, "PageEnb"=T3."Page Disabled & Grayed" ("Page Enabled State")) -> ()  [unwired: 1 in, 2 out]
            n265 = property class="Page"(reference=w363, "PageEnb"=T3."Page Disabled & Grayed" ("Page Enabled State")) -> ()  [unwired: 1 in, 2 out]
            n266 = property class="Str"("Value"="  ") -> ()  [unwired: 2 in, 2 out]
          }
          event "Add User": Value Change {
            n267 = event-data() -> ()  [unwired: 1 in, 6 out]
            n268 = property on="Tab Control" class="TabCtl (strict)"("Value"=T1."Add User" ("Tab Control")) -> ()  [unwired: 2 in, 2 out]
            n269 = property on="Userdata_add_page" class="Clust (strict)"("Value"=T2 {"Username"="", "Password"="", "Title"="", "Birthdate"=timestamp(0 s since 1904-01-01), "Email"="", "User Level"=FALSE} ("Userdata_add_page")) -> ()  [unwired: 2 in, 2 out]
            n270 = property on="Tab Control" class="TabCtl (strict)"() -> ("Pages"=w371:refnum<vi>[])  [unwired: 2 in, 2 out]
            n271 = Index Array(array=w371, index=2) -> (element=w370:refnum<vi>)
            n272 = property class="Page"(reference=w370, "PageEnb"=T3."Page Enabled" ("Page Enabled State")) -> ()  [unwired: 1 in, 2 out]
          }
          event "Delete User": Value Change {
            n273 = event-data() -> ()  [unwired: 1 in, 6 out]
            n274 = property on="Tab Control" class="TabCtl (strict)"("Value"=T1."Delete User" ("Tab Control")) -> ()  [unwired: 2 in, 2 out]
            n275 = property on="Userdata_delete_page" class="Clust (strict)"("Value"=T2 {"Username"="", "Password"="", "Title"="", "Birthdate"=timestamp(0 s since 1904-01-01), "Email"="", "User Level"=FALSE} ("Userdata_add_page")) -> ()  [unwired: 2 in, 2 out]
            n276 = property on="Tab Control" class="TabCtl (strict)"() -> ("Pages"=w376:refnum<vi>[])  [unwired: 2 in, 2 out]
            n277 = Index Array(array=w376, index=3) -> (element=w377:refnum<vi>)
            n278 = property class="Page"(reference=w377, "PageEnb"=T3."Page Enabled" ("Page Enabled State")) -> ()  [unwired: 1 in, 2 out]
          }
          event "Query User": Value Change {
            n279 = event-data() -> ()  [unwired: 1 in, 6 out]
            n280 = property on="Tab Control" class="TabCtl (strict)"() -> ("Pages"=w382:refnum<vi>[])  [unwired: 2 in, 2 out]
            n281 = property on="Tab Control" class="TabCtl (strict)"("Value"=T1."Query User" ("Tab Control")) -> ()  [unwired: 2 in, 2 out]
            n282 = Index Array(array=w382, index=4) -> (element=w383:refnum<vi>)
            n283 = property on="Userdata_Query_page" class="Clust (strict)"("Value"=T2 {"Username"="", "Password"="", "Title"="", "Birthdate"=timestamp(0 s since 1904-01-01), "Email"="", "User Level"=FALSE} ("Userdata_add_page")) -> ()  [unwired: 2 in, 2 out]
            n284 = property class="Page"(reference=w383, "PageEnb"=T3."Page Enabled" ("Page Enabled State")) -> ()  [unwired: 1 in, 2 out]
          }
          event "Edit User": Value Change {
            n285 = event-data() -> ()  [unwired: 1 in, 6 out]
            n286 = property on="Tab Control" class="TabCtl (strict)"("Value"=T1."Edit User" ("Tab Control")) -> ()  [unwired: 2 in, 2 out]
            n287 = property on="Userdata_Edit_page" class="Clust (strict)"("Value"=T2 {"Username"="", "Password"="", "Title"="", "Birthdate"=timestamp(0 s since 1904-01-01), "Email"="", "User Level"=FALSE} ("Userdata_add_page")) -> ()  [unwired: 2 in, 2 out]
            n288 = property on="Tab Control" class="TabCtl (strict)"() -> ("Pages"=w388:refnum<vi>[])  [unwired: 2 in, 2 out]
            n289 = Index Array(array=w388, index=5) -> (element=w389:refnum<vi>)
            n290 = property class="Page"(reference=w389, "PageEnb"=T3."Page Enabled" ("Page Enabled State")) -> ()  [unwired: 1 in, 2 out]
          }
          event "Exit", "Exit 2": Value Change {
            n291 = event-data() -> ()  [unwired: 1 in, 6 out]
          }
        }
      }
    }
  }
